vi "Update Stations.vi"(8 "error in (no error)":errorcluster, 10 "Combo Value":string, 11 "OPC Server in":refnum<class "OPC Server.lvclass">) -> (0 "error out":errorcluster, 3 "OPC Server out":refnum<class "OPC Server.lvclass">)   [LabVIEW 2021, in "OPC Server.lvlib" / "OPC Server.lvclass"]
uses:
  OPC Server.lvclass
  OPC Server.lvclass/OPC Server.ctl
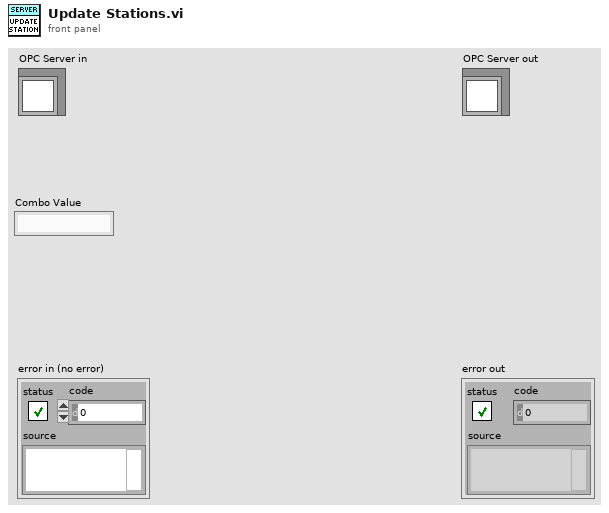
[diagram p1: front panel]
types:
  T1 = map{string, refnum<class "Message Enqueuer.lvclass">}
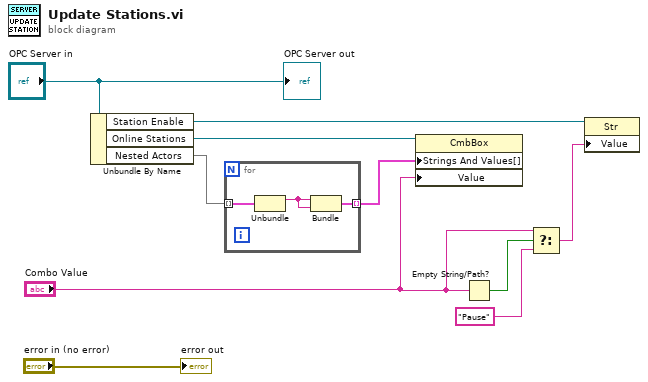
[diagram p0: block diagram]
diagram:
  n1 = Unbundle By Name("OPC Server in") -> ("Station Enable"=w5:refnum<vi>, "Online Stations"=w9:refnum<vi>, "Nested Actors"=w8:T1)
  n2 = for {
    tunnel: w8 -> [w13] mode=indexing
    tunnel: [w11] -> w7 mode=indexing
    n3 = Unbundle(w13) -> (w12:string)  [unwired: 1 out]
    n4 = Bundle(w12, w12) -> (w11:cluster{string, string})  [unwired: 1 in]
  }
  n5 = property class="CmbBox"(reference=w9, "Strings And Values[]"=w7, "Value"="Combo Value") -> ()  [unwired: 1 in, 2 out]
  n6 = Empty String/Path?(string/path="Combo Value") -> (empty?=w4:bool)
  n7 = Select(t="Combo Value", s=w4, f="Pause") -> (s? t:f=w1:string)
  n8 = property class="Str"(reference=w5, "Value"=w1) -> ()  [unwired: 1 in, 2 out]
  "error out" <- "error in (no error)"
  "OPC Server out" <- "OPC Server in"
